vi "CheckIfFileExists.vi"(8 "error in (no error)":errorcluster, 11 "path":path) -> (0 "error out":errorcluster, 2 "file\\folder exists?":bool, 3 "dup path":path)   [LabVIEW 2017, in "USBDrive.lvlib"]
doc: "Checks whether a file or folder exists on disk at a specified path. This VI works with standard files and folders as well as files in LLB files."
uses:
  <vilib>/addons/InsightCM/Devices/Shared/Common/USBDrive/USBDrive.lvlib
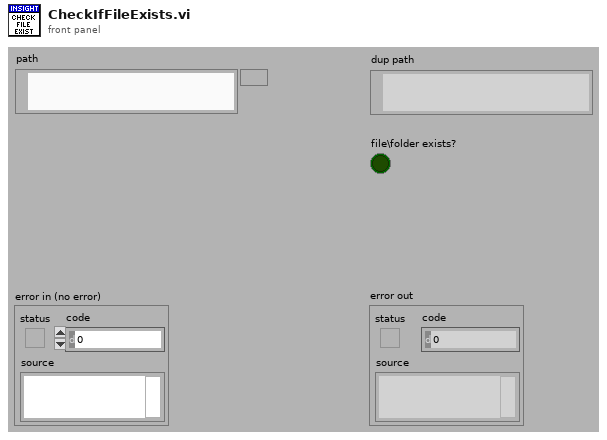
[diagram p1: front panel]
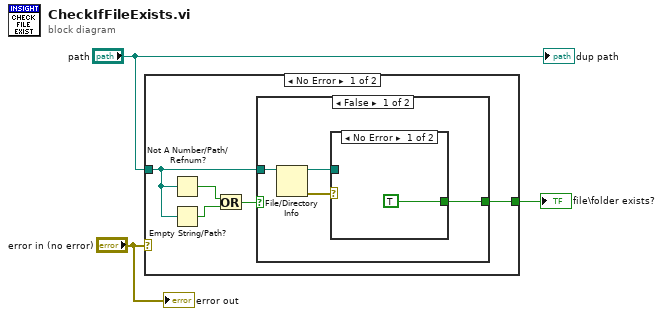
[diagram p0: block diagram]
diagram:
  n1 = case shown="No Error" "error in (no error)" {
    tunnel: "path" -> [w4 _]
    tunnel: [w8 _] -> w3
    frame No Error {
      n2 = Not A Number/Path/Refnum?(number/path/refnum=w4) -> (NaN/Path/Refnum?=w7:bool)
      n3 = Empty String/Path?(string/path=w4) -> (empty?=w6:bool)
      n4 = Or(x=w7, y=w6) -> (x .or. y?=w5:bool)
      n5 = case shown="False" w5 {
        tunnel: [w10 _] -> w8
        tunnel: w4 -> [w12 _]
        frame False {
          n6 = File/Directory Info(path=w12) -> (path out=w9:path, error out=w11:errorcluster)  [unwired: 1 in, 5 out]
          n7 = case shown="No Error" w11 {
            tunnel: [TRUE _] -> w10
            tunnel: w9 -> [_ _]
            frame No Error {
            }
            frame Error {
            }
          }
        }
        frame True {
        }
      }
    }
    frame Error {
    }
  }
  "file\\folder exists?" <- w3
  "error out" <- "error in (no error)"
  "dup path" <- "path"
